vi "Select ROIs.vi"(8 "error in (no error)":errorcluster, 11 "Retiga in":refnum<class "Retiga.lvclass">) -> (0 "error out":errorcluster, 3 "Retiga out":refnum<class "Retiga.lvclass">)   [LabVIEW 2012, in "Retiga.lvclass"]
uses:
  Retiga.lvclass
  Retiga.lvclass/Retiga.ctl
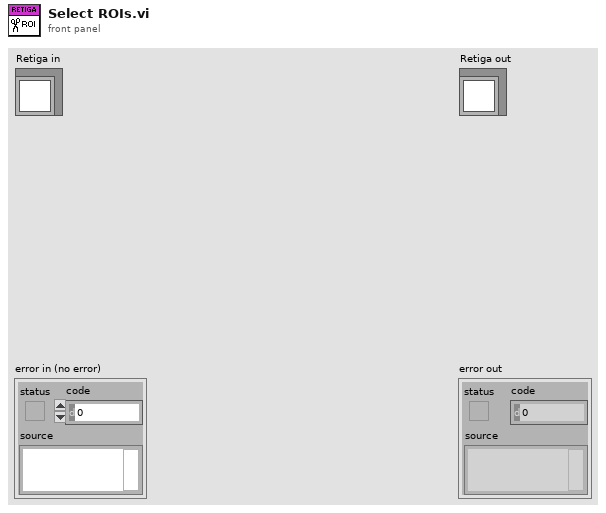
[diagram p1: front panel]
types:
  T1 = typedef "IMAQ Rectangle" = cluster{"Left":i32, "Top":i32, "Right":i32, "Bottom":i32, "Rotation":dbl}
  T2 = typedef "IMAQ Image.ctl" = refnum<image>
  T3 = typedef "ROI Descriptor" = cluster{"Global Rectangle":i32[], "Contours":cluster{"ID":enum32{"External", "Internal"}, "Type":u32, "Coordinates":i32[]}[]}
  T4 = cluster{"[0]":i32, "[1]":i32, "[2]":i32, "[3]":i32, "[4]":i32, "[5]":i32, "[6]":i32, "[7]":i32, "[8]":i32}
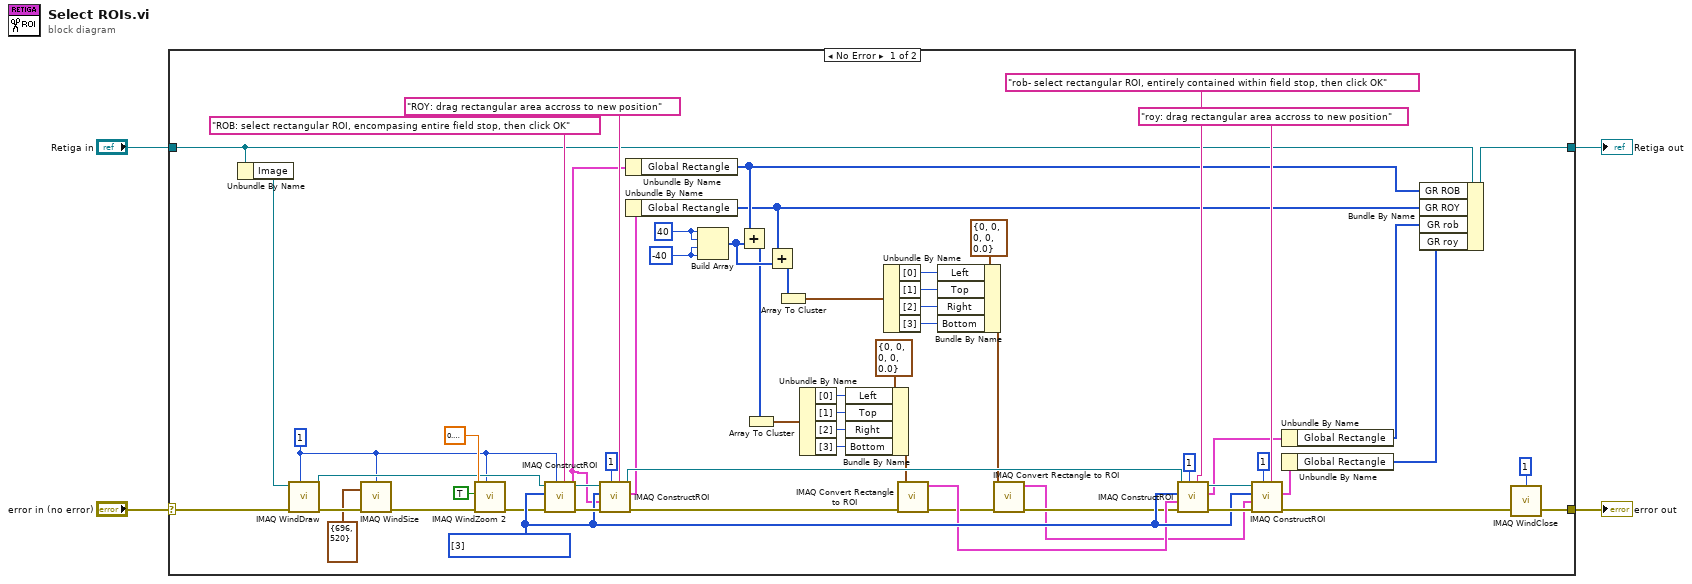
[diagram p0: block diagram]
diagram:
  n1 = case shown="No Error" "error in (no error)" {
    selector: "error in (no error)" -> [w7 w66]
    tunnel: [w6 w66] -> w3
    tunnel: [w5 w65] -> w1
    tunnel: "Retiga in" -> [w8 w65]
    frame No Error {
      w35 = -40
      w36 = 40
      w38 = 1 ("Window Number (0...15)")
      w51 = u32[] [3] items=["No Selection", "Point", "Line", "Rectangle", "Oval", "Polygon", "Freehand Region", "Annulus", "Zoom", "Pan", "Broken Line", "Freehand Line", "Rotated Rectangle"] ("Tools")
      n2 = Unbundle By Name(w8) -> ("Image"=w61:T2)
      n3 = call "IMAQ WindDraw"("Window Number (0...15)"=w38, "error in (no error)"=w7, "Image"=w61) -> ("error out"=w40:errorcluster, "Image Out (duplicate)"=w63:T2)  [unwired: 7 in]
      n4 = call "IMAQ WindSize"("error in (no error)"=w40, "Width & Height"=cluster{"Width":i32, "Height":i32} {"Width"=696, "Height"=520}, "Window Number"=w38) -> ("error out"=w39:errorcluster)  [unwired: 3 in, 2 out]
      n5 = call "IMAQ WindZoom 2"("Window Number (0...15)"=w38, "error in (no error)"=w39, "Zoom to Fit? (False)"=TRUE, "Zoom Factor"=sgl 0.9) -> ("error out"=w41:errorcluster)  [unwired: 4 in, 3 out]
      n6 = call "IMAQ ConstructROI"("Prompt"="ROB: select rectangular ROI, encompasing entire field stop, then click OK", "Window Number (-1...15)"=w38, "error in (no error)"=w41, "Tools"=w51, "Image"=w63) -> ("error out"=w58:errorcluster, "ROI Descriptor Out"=w31:T3, "Image Out (duplicate)"=w57:T2)  [unwired: 3 in, 1 out]
      n7 = call "IMAQ ConstructROI"("Prompt"="ROY: drag rectangular area accross to new position", "Window Number (-1...15)"=1, "error in (no error)"=w58, "ROI Descriptor In (None)"=w31, "Tools"=w51, "Image"=w57) -> ("error out"=w19:errorcluster, "ROI Descriptor Out"=w30:T3, "Image Out (duplicate)"=w53:T2)  [unwired: 2 in, 1 out]
      n8 = Unbundle By Name(w31) -> ("Global Rectangle"=w34:i32[])
      n9 = Unbundle By Name(w30) -> ("Global Rectangle"=w33:i32[])
      n10 = Build Array(w36, w36, w35, w35) -> (w32:i32[])
      n11 = Add(x=w34, y=w32) -> (x+y=w28:i32[])
      n12 = Array To Cluster(array=w28) -> (cluster=w27:T4)
      n13 = Add(x=w33, y=w32) -> (x+y=w16:i32[])
      n14 = Array To Cluster(array=w16) -> (cluster=w15:T4)
      n15 = Unbundle By Name(w27) -> ("[0]"=w26:i32, "[1]"=w25:i32, "[2]"=w24:i32, "[3]"=w23:i32)
      n16 = Bundle By Name(cluster=T1 {"Left"=0, "Top"=0, "Right"=0, "Bottom"=0, "Rotation"=0.0} ("Rectangle"), "Left"=w26, "Top"=w25, "Right"=w24, "Bottom"=w23) -> (w22:T1)
      n17 = Unbundle By Name(w15) -> ("[0]"=w14:i32, "[1]"=w13:i32, "[2]"=w12:i32, "[3]"=w11:i32)
      n18 = call "IMAQ Convert Rectangle to ROI"("error in (no error)"=w19, "Rectangle"=w22) -> ("error out"=w20:errorcluster, "ROI Descriptor"=w21:T3)  [unwired: 7 in]
      n19 = Bundle By Name(cluster=T1 {"Left"=0, "Top"=0, "Right"=0, "Bottom"=0, "Rotation"=0.0} ("Rectangle"), "Left"=w14, "Top"=w13, "Right"=w12, "Bottom"=w11) -> (w10:T1)
      n20 = call "IMAQ Convert Rectangle to ROI"("error in (no error)"=w20, "Rectangle"=w10) -> ("error out"=w18:errorcluster, "ROI Descriptor"=w9:T3)  [unwired: 7 in]
      n21 = call "IMAQ ConstructROI"("Prompt"="rob- select rectangular ROI, entirely contained within field stop, then click OK", "Window Number (-1...15)"=1, "error in (no error)"=w18, "ROI Descriptor In (None)"=w21, "Tools"=w51, "Image"=w53) -> ("error out"=w54:errorcluster, "ROI Descriptor Out"=w42:T3, "Image Out (duplicate)"=w52:T2)  [unwired: 2 in, 1 out]
      n22 = call "IMAQ ConstructROI"("Prompt"="roy: drag rectangular area accross to new position", "Window Number (-1...15)"=1, "error in (no error)"=w54, "ROI Descriptor In (None)"=w9, "Tools"=w51, "Image"=w52) -> ("error out"=w48:errorcluster, "ROI Descriptor Out"=w50:T3)  [unwired: 2 in, 2 out]
      n23 = Unbundle By Name(w42) -> ("Global Rectangle"=w47:i32[])
      n24 = Unbundle By Name(w50) -> ("Global Rectangle"=w46:i32[])
      n25 = Bundle By Name(cluster=w8, "GR ROB"=w34, "GR ROY"=w33, "GR rob"=w47, "GR roy"=w46) -> (w5:refnum<class "Retiga.lvclass">)
      n26 = call "IMAQ WindClose"("Window Number (0...15)"=1, "error in (no error)"=w48) -> ("error out"=w6:errorcluster)  [unwired: 4 in]
    }
    frame Error {
    }
  }
  "error out" <- w3
  "Retiga out" <- w1
